vi "ELVIS III v1.1 Open AO (N Samples).vi"(7 "Allow multiple opens?":bool, 8 "error in (no error)":errorcluster, 10 "Channel Names":string[](array[string]), 11 "Resource name":T5 caption="RIO Device") -> (0 "error out":errorcluster, 1 "AO (N Samples) Scale Constants List":T1, 2 "AO (N Samples) Channel List":T6, 3 "myRIO Ref Out":T3)   [LabVIEW 2021]
uses:
  <vilib>/myRIO/Common/Instrument Driver Framework/myRIO v1.0/AO Block/typedefs/AO Block Channels List.ctl
  <vilib>/myRIO/Common/Instrument Driver Framework/myRIO v1.0/AO Block/typedefs/AO Block Channels Enum.ctl
  <vilib>/userDefined/High Color/nirio_resource_hc.ctl
  <vilib>/myRIO/Common/Instrument Driver Framework/Utilities/typedefs/myRIO v1.0 Reference.ctl
  <vilib>/myRIO/Common/Instrument Driver Framework/Utilities/typedefs/Generic FPGA Reference.ctl
  <vilib>/myRIO/Common/Instrument Driver Framework/Utilities/typedefs/Analog Scaling Constants List.ctl
  <vilib>/myRIO/Common/Instrument Driver Framework/Utilities/typedefs/Analog Scaling Constants.ctl
  <vilib>/myRIO/Common/Instrument Driver Framework/ELVIS III v1.0/AO Block/typedefs/ELVIS III v1.0 AO Block Channels Enum.ctl
  <vilib>/Utility/VariantDataType/GetNumericInfo.vi
  <vilib>/Utility/error.llb/Error Cluster From Error Code.vi
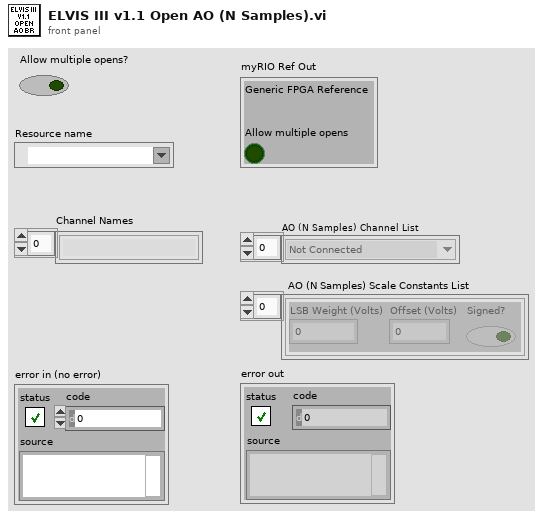
[diagram p1: front panel]
types:
  T1 = typedef "Analog Scaling Constants List.ctl" = T2[]
  T2 = typedef "Analog Scaling Constants.ctl" = cluster{"LSB Weight (Volts)":dbl, "Offset (Volts)":dbl, "Signed?":bool}
  T3 = typedef "myRIO v1.0 Reference.ctl" = cluster{"Generic FPGA Reference":T4, "Allow multiple opens":bool}
  T4 = typedef "Generic FPGA Reference.ctl" = refnum<k20>
  T5 = typedef "nirio_resource_hc.ctl" = tag
  T6 = typedef "AO Block Channels List.ctl" = T7[]
  T7 = typedef "AO Block Channels Enum.ctl" = enum16{"Not Connected", "A/AO0 (N Samples)", "A/AO1 (N Samples)", "B/AO0 (N Samples)", "B/AO1 (N Samples)"}
  T8 = typedef "ELVIS III v1.0 AO Block Channels Enum.ctl" = enum16{"Not Connected", "A/AO0 (N Samples)", "A/AO1 (N Samples)", "B/AO0 (N Samples)", "B/AO1 (N Samples)"}
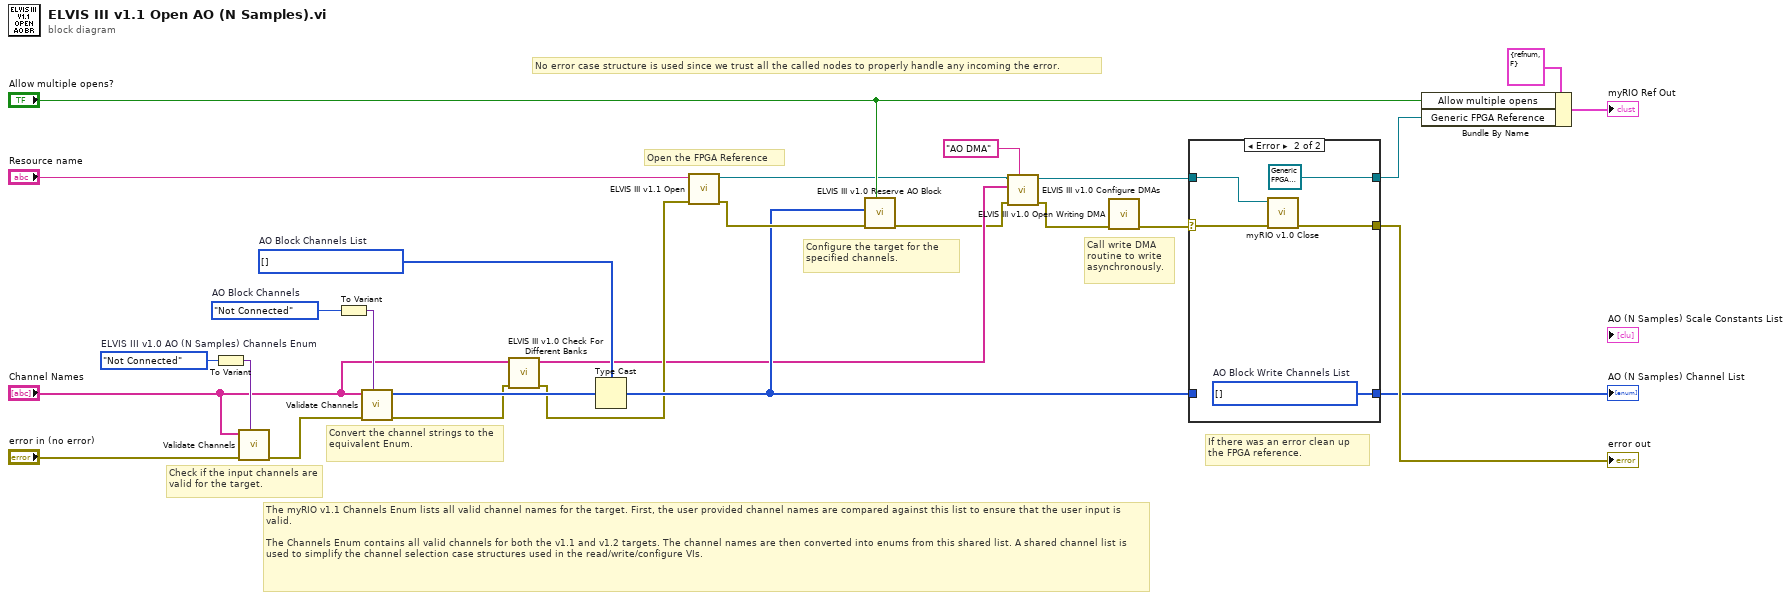
[diagram p0: block diagram]
diagram:
  w12 = T6 [] items=["Not Connected", "A/AO0 (N Samples)", "A/AO1 (N Samples)", "B/AO0 (N Samples)", "B/AO1 (N Samples)"]  # AO Block Channels List
  w13 = AO_Block_Channels_Enum."Not Connected"  # AO Block Channels
  w14 = ELVIS_III_v1.0_AO_Block_Channels_Enum."Not Connected"  # ELVIS III v1.0 AO (N Samples) Channels Enum
  # "Call write DMA\nroutine to write \nasynchronously."
  # "The myRIO v1.1 Channels Enum lists all valid channel names for the target. First, the user provided channel names are compared against this list to ensure that the user input is valid.\n\nThe Channels Enum contains all valid channels for both the v1.1 and v1.2 targets. The channel names are then converted into enums from this shared list. A shared channel list is used to simplify the channel selection case structures used in the read/write/configure VIs."
  # "If there was an error clean up the FPGA reference."
  # "Configure the target for the specified channels."
  # "Open the FPGA Reference"
  # "No error case structure is used since we trust all the called nodes to properly handle any incoming the error."
  # "Convert the channel strings to the equivalent Enum."
  # "Check if the input channels are valid for the target."
  n1 = To Variant(anything=w14) -> (Variant=w17:variant)
  n2 = call <vilib>:"Validate Channels.vi"("Channels Enum Variant"=w17, "error in (no error)"="error in (no error)", "Channel Names"="Channel Names") -> ("error out"=w25:errorcluster)  [unwired: 7 in, 1 out]
  n3 = To Variant(anything=w13) -> (Variant=w18:variant)
  n4 = call <vilib>:"Validate Channels.vi"("Channels Enum Variant"=w18, "error in (no error)"=w25, "Channel Names"="Channel Names") -> ("error out"=w8:errorcluster, "Index Array"=w22:u16[])  [unwired: 7 in]
  n5 = call <vilib>:"ELVIS III v1.0 Check For Different Banks.vi"("error in (no error)"=w8, "Channel Names"="Channel Names") -> ("error out"=w7:errorcluster)  [unwired: 9 in]
  n6 = Type Cast(type=w12, x=w22) -> (*(type *) &x=w9:T6)
  n7 = call <vilib>:"ELVIS III v1.1 Open.vi"("error in (no error)"=w7, "Resource name"="Resource name") -> ("error out"=w10:errorcluster, "myRIO FPGA Ref Out"=w6:T4)  [unwired: 8 in]
  n8 = call <vilib>:"ELVIS III v1.0 Reserve AO Block.vi"("Allow multiple opens?"="Allow multiple opens?", "error in (no error)"=w10, "AO (N Samples) Channel List"=w9) -> ("error out"=w3:errorcluster)  [unwired: 8 in]
  n9 = call <vilib>:"ELVIS III v1.0 Configure DMAs.vi"("DMA Type"="AO DMA", "error in (no error)"=w3, "Channel Names"="Channel Names", "ELVIS III FPGA Ref"=w6) -> ("error out"=w2:errorcluster, "ELVIS III FPGA Ref"=w5:T4)  [unwired: 6 in]
  n10 = call <vilib>:"ELVIS III v1.0 Open Writing DMA.vi"("error in (no error)"=w2) -> ("error out"=w11:errorcluster)  [unwired: 10 in]
  n11 = case shown="Error" w11 {
    selector: w11 -> [w29 w34]
    tunnel: w5 -> [w27 w32]
    tunnel: [w27 T4 refnum ("myRIO FPGA Ref Out")] -> w19
    tunnel: [w29 w33] -> w23
    tunnel: w9 -> [w28 _]
    tunnel: [w28 w30] -> w21
    frame No Error {
    }
    frame Error {
      w30 = T6 [] items=["Not Connected", "A/AO0 (N Samples)", "A/AO1 (N Samples)", "B/AO0 (N Samples)", "B/AO1 (N Samples)"]  # AO Block Write Channels List
      n12 = call <vilib>:"myRIO v1.0 Close.vi"("error in (no error)"=w34, "myRIO FPGA Ref In"=w32) -> ("error out"=w33:errorcluster)  [unwired: 9 in]
    }
  }
  "AO (N Samples) Channel List" <- w21
  "error out" <- w23
  n13 = Bundle By Name(cluster=T3 {"Generic FPGA Reference"=refnum, "Allow multiple opens"=FALSE} ("myRIO Ref Out"), "Allow multiple opens"="Allow multiple opens?", "Generic FPGA Reference"=w19) -> (→"myRIO Ref Out":T3)
